vi "Caller Notice.vi"(8 "error in (no error)":errorcluster, 9 "Params":variant, 10 "Action Name":string, 11 "Generic Actor in":refnum<class "Generic Actor.lvclass">) -> (0 "error out":errorcluster, 3 "Generic Actor out":refnum<class "Generic Actor.lvclass">)   [LabVIEW 2020, in "Generic Actor.lvlib" / "Generic Actor.lvclass"]
uses:
  Generic Actor.lvclass
  C:/Program Files (x86)/National Instruments/LabVIEW 2020/vi.lib/ActorFramework/Actor/Actor.lvclass
  <vilib>/ActorFramework/Actor/Actor.lvclass/Actor.ctl
  Generic Actor.lvclass/Generic Actor.ctl
  Generic Actor Messages/Caller Notice Msg/Caller Notice Msg.lvclass/Caller Notice Msg.ctl
  <vilib>/ActorFramework/Message Enqueuer/Message Enqueuer.lvclass/Message Enqueuer.ctl
  <vilib>/ActorFramework/Message Enqueuer/Enqueue.vi
  Generic Actor Messages/Caller Notice Msg/Caller Notice Msg.lvclass
  C:/Program Files (x86)/National Instruments/LabVIEW 2020/vi.lib/ActorFramework/Message/Message.lvclass
  <vilib>/ActorFramework/Message Priority Queue/Priority Enqueue.vi
  <vilib>/ActorFramework/Actor/Actor.lvclass
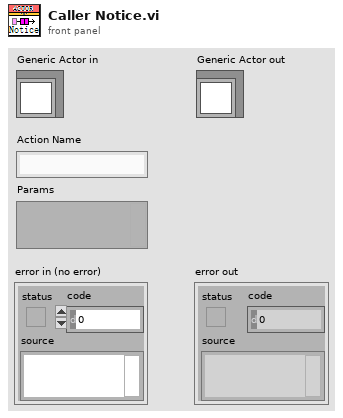
[diagram p1: front panel]
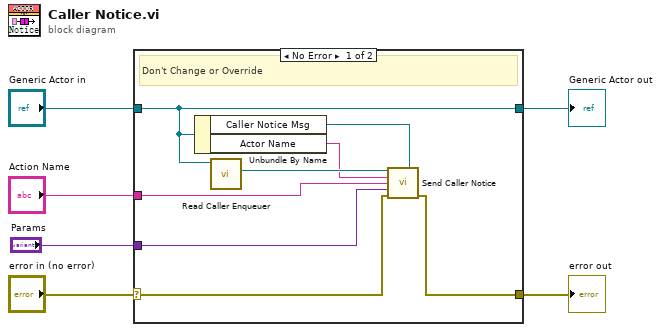
[diagram p0: block diagram]
diagram:
  n1 = case shown="No Error" "error in (no error)" {
    selector: "error in (no error)" -> [w11 w16]
    tunnel: [w10 w16] -> w5
    tunnel: [w9 w15] -> w3
    tunnel: "Generic Actor in" -> [w9 w15]
    tunnel: "Action Name" -> [w13 _]
    tunnel: "Params" -> [w12 _]
    frame No Error {
      # "Don't Change or Override"
      n2 = Unbundle By Name(w9) -> ("Caller Notice Msg"=w8:refnum<class "Caller Notice Msg.lvclass">, "Actor Name"=w7:string)
      n3 = call <vilib>:"Read Caller Enqueuer.vi"("Actor"=w9) -> ("Caller Enqueuer"=w14:refnum<class "Message Enqueuer.lvclass">)  [unwired: 10 in]
      n4 = call "Send Caller Notice .vi"("Message Enqueuer"=w14, "Message Type"=w8, "Actor Name"=w7, "Action Name"=w13, "Params"=w12, "error in (no error)"=w11) -> ("error out"=w10:errorcluster)  [unwired: 8 in, 1 out]
    }
    frame Error {
    }
  }
  "error out" <- w5
  "Generic Actor out" <- w3
